vi "UT_008_Get TOML data.vi"   [LabVIEW 2017]
uses:
  <vilib>/addons/_JKI Toolkits/Caraya/classes/Assert/Assert True.vi
  <vilib>/addons/_JKI Toolkits/Caraya/classes/Assert/Assert Equal Value_Variant.vi
  <vilib>/addons/_JKI Toolkits/Caraya/classes/Test/Test.lvclass
  <vilib>/addons/_JKI Toolkits/Caraya/classes/Assert/Assert.lvclass
  lib/TOML.lvlib
types:
  T1 = cluster{"cluster":cluster{"string":string, "bool":bool, "path":path}, "1d-array-cluster":cluster{"string":string, "int":i32}[]}
  T2 = cluster{"string":string, "bool":bool, "path":path}
  T3 = typedef "TOML.lvlib/TOML Value.ctl" = cluster{"type":enum16{"Table", "Array", "String", "Integer", "Float", "Boolean", "Offset Date-Time", "Local Date-Time", "Local Date", "Local Time", "Path"}, "value":variant}
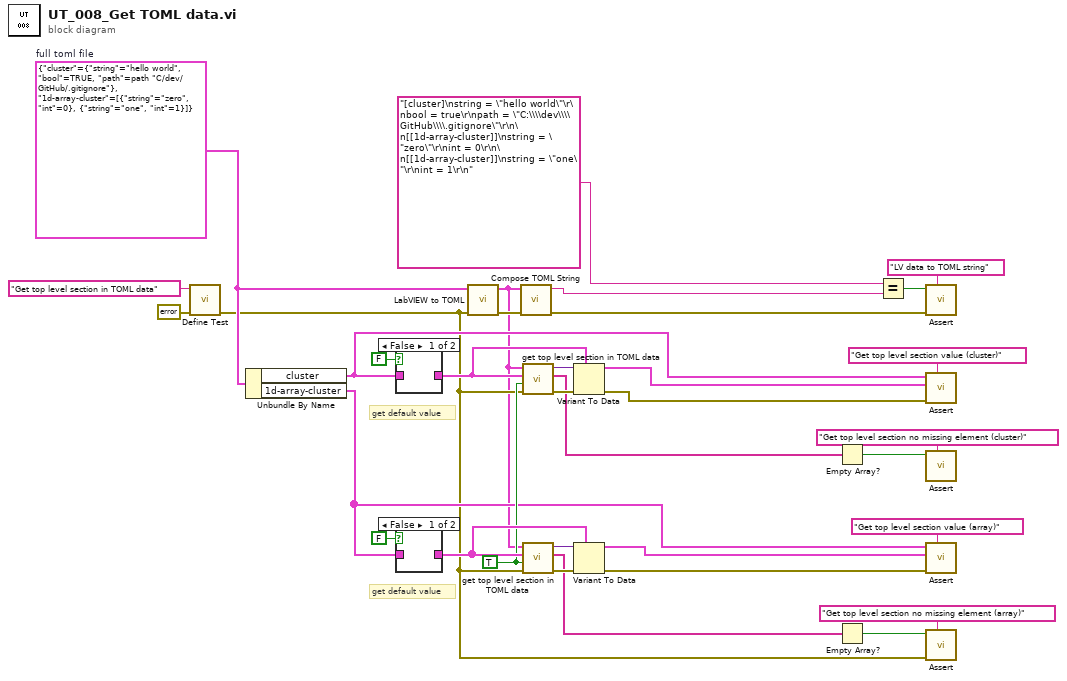
[diagram p0: block diagram]
diagram:
  w7 = TRUE ("Error if missing element")
  w23 = T1 {"cluster"={"string"="hello world", "bool"=TRUE, "path"=path "C:/dev/GitHub/.gitignore"}, "1d-array-cluster"=[{"string"="zero", "int"=0}, {"string"="one", "int"=1}]}  # full toml file
  # "get default value"
  # "get default value"
  n1 = call <vilib>:"Define Test.vi"("error in (no error)"=errorcluster {"status"=FALSE, "code"=0, "source"=""}, "Label (VI Title)"="Get top level section in TOML data") -> ("error out"=w3:errorcluster)  [unwired: 9 in]
  n2 = Unbundle By Name(w23) -> ("cluster"=w18:T2, "1d-array-cluster"=w6:cluster{"string":string, "int":i32}[])
  n3 = case shown="False" FALSE {
    tunnel: [_ w35] -> w16
    tunnel: w18 -> [_ w35]
    frame False {
    }
    frame True {
    }
  }
  n4 = case shown="False" FALSE {
    tunnel: [_ w36] -> w12
    tunnel: w6 -> [_ w36]
    frame False {
    }
    frame True {
    }
  }
  n5 = call "LabVIEW to TOML.vi"("error in (no error)"=w3, "LV Value"=w23) -> ("error out"=w27:errorcluster, "TOML Value"=w1:T3)  [unwired: 7 in, 1 out]
  n6 = call "Compose TOML String.vi"("error in (no error)"=w27, "Value"=w1) -> ("error out"=w26:errorcluster, "String"=w25:string)  [unwired: 8 in]
  n7 = call "get top level section in TOML data.vi"("error in (no error)"=w3, "Error if missing element"=w7, "Section datatype"=w16, "Value in"=w1) -> ("error out"=w21:errorcluster, "Missing elements"=w15:string[], "LV Value"=w20:variant)  [unwired: 5 in]
  n8 = call "get top level section in TOML data.vi"("error in (no error)"=w3, "Error if missing element"=w7, "Section datatype"=w12, "Value in"=w1) -> ("error out"=w10:errorcluster, "Missing elements"=w4:string[], "LV Value"=w11:variant)  [unwired: 5 in]
  n9 = Variant To Data(error in=w21, type=w16, Variant=w20) -> (data=w17:T2, error out=w19:errorcluster)
  n10 = Variant To Data(error in=w10, type=w12, Variant=w11) -> (data=w5:cluster{"string":string, "int":i32}[], error out=w8:errorcluster)
  n11 = Empty Array?(array=w15) -> (empty?=w14:bool)
  n12 = Empty Array?(array=w4) -> (empty?=w2:bool)
  n13 = Equal?(x="[cluster]\nstring = \"hello world\"\r\nbool = true\r\npath = \"C:\\\\dev\\\\GitHub\\\\.gitignore\"\r\n\n[[1d-array-cluster]]\nstring = \"zero\"\r\nint = 0\r\n\n[[1d-array-cluster]]\nstring = \"one\"\r\nint = 1\r\n", y=w25) -> (x = y?=w29:bool)
  n14 = call-poly <vilib>:"Assert.vi"("Label"="LV data to TOML string" ("Label (VI Title)"), "error in (no error)"=w26, "True?"=w29) -> ()  [unwired: 8 in, 1 out]
  n15 = call-poly <vilib>:"Assert.vi"("Label"="Get top level section value (cluster)" ("Label (VI Title)"), "error in (no error)"=w19, "Y"=w17, "X"=w18) -> ()  [unwired: 7 in, 1 out]
  n16 = call-poly <vilib>:"Assert.vi"("Label"="Get top level section no missing element (cluster)" ("Label (VI Title)"), "True?"=w14) -> ()  [unwired: 9 in, 1 out]
  n17 = call-poly <vilib>:"Assert.vi"("Label"="Get top level section value (array)" ("Label (VI Title)"), "error in (no error)"=w8, "Y"=w5, "X"=w6) -> ()  [unwired: 7 in, 1 out]
  n18 = call-poly <vilib>:"Assert.vi"("Label"="Get top level section no missing element (array)" ("Label (VI Title)"), "error in (no error)"=w3, "True?"=w2) -> ()  [unwired: 8 in, 1 out]
